vi "Queued State Machine.vi"() -> ()   [LabVIEW 2009]
doc: "Ce VI est un modèle de machine à états basée sur une file d'attente. Remplacez Processus 1 et Processus 2 par vos états. Pour ajouter d'autres processus, modifiez la constante énumération à définition de type. L'ordre de l'énumération doit correspondre à celui du cluster."
uses:
  Queued State Enum.ctl
panel:
  in  "Menu":T1
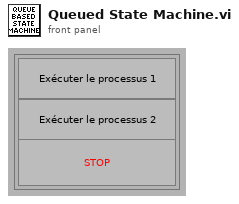
[diagram p1: front panel]
types:
  T1 = cluster{"Processus 1":bool, "Processus 2":bool, "stop":bool}
  T2 = typedef "Queued State Enum.ctl" = enum32{"Inactif", "Processus 1", "Processus 2", "Arrêt"}
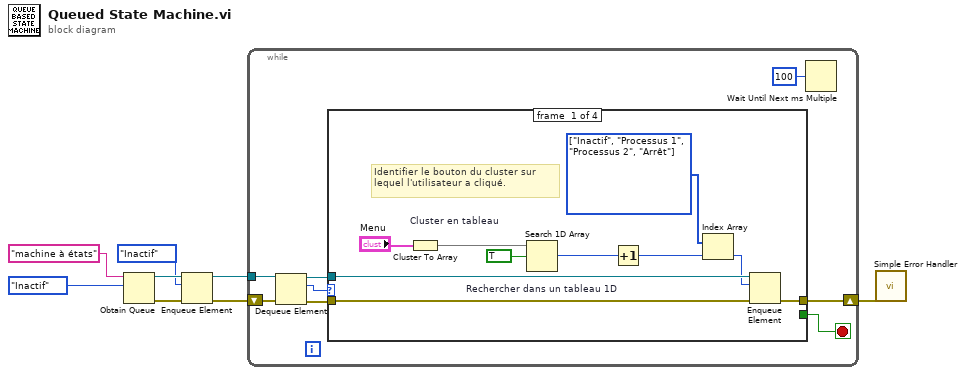
[diagram p0: block diagram]
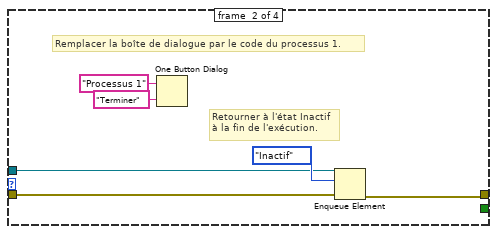
[diagram p2: hidden frame]
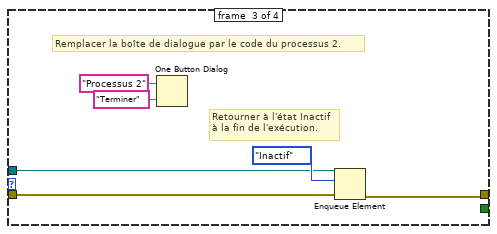
[diagram p3: hidden frame]
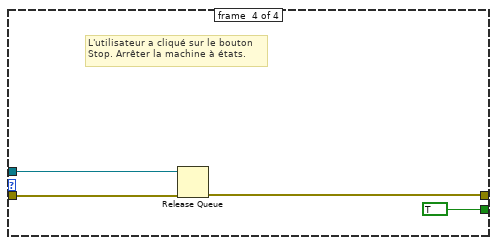
[diagram p4: hidden frame]
diagram:
  n1 = Obtain Queue ("Obtenir une file d'attente")(name (unnamed)="machine à états", element data type=Queued_State_Enum."Inactif" ("Enum")) -> (queue out=w6:refnum<queue>, error out=w7:errorcluster)  [unwired: 3 in, 1 out]
  n2 = Enqueue Element ("Ajouter un élément à la fin d'une file d'attente")(queue=w6, element=Queued_State_Enum."Inactif" ("Enum"), error in (no error)=w7) -> (queue out=w4:refnum<queue>, error out=w5:errorcluster)  [unwired: 2 out]
  n3 = while "Boucle While" {
    tunnel: w4 -> [w11]
    shift-right: [w14] -> w1
    shift-left: w5 -> [w13]
    stop <- w16 stop-if-true
    n4 = Dequeue Element ("Supprimer le premier élément d'une file d'attente")(queue=w11, error in (no error)=w13) -> (queue out=w10:refnum<queue>, element=w9:T2, error out=w12:errorcluster)  [unwired: 2 out]
    n5 = case "Structure Condition" shown="\"Inactif\", Par défaut" w9 {
      tunnel: [_ _ _ TRUE] -> w16
      tunnel: w12 -> [w22 w30 w36 w41]
      tunnel: w10 -> [w21 w27 w33 w40]
      tunnel: [w20 w29 w35 w39] -> w14
      frame #0 {
        w18 = T2[] [enum."Inactif", enum."Processus 1", enum."Processus 2", enum."Arrêt"] items=["Inactif", "Processus 1", "Processus 2", "Arrêt"]
        # "Identifier le bouton du cluster sur lequel l'utilisateur a cliqué."
        n6 = Cluster To Array "Cluster en tableau"(cluster="Menu") -> (array=w25:bool[])
        n7 = Search 1D Array "Rechercher dans un tableau 1D"(1D array=w25, element=TRUE) -> (index of element=w23:i32)  [unwired: 1 in]
        n8 = Increment(x=w23) -> (x+1=w19:i32)
        n9 = Index Array(array=w18, index=w19) -> (element=w17:T2)
        n10 = Enqueue Element(queue=w21, element=w17, error in (no error)=w22) -> (error out=w20:errorcluster)  [unwired: 3 out]
      }
      frame #1 {
        # "Retourner à l'état Inactif\nà la fin de l'exécution."
        # "Remplacer la boîte de dialogue par le code du processus 1."
        n11 = One Button Dialog(message="Processus 1", button name ("OK")="Terminer") -> ()  [unwired: 1 out]
        n12 = Enqueue Element(queue=w27, element=Queued_State_Enum."Inactif" ("Enum"), error in (no error)=w30) -> (error out=w29:errorcluster)  [unwired: 3 out]
      }
      frame #2 {
        # "Retourner à l'état Inactif\nà la fin de l'exécution."
        # "Remplacer la boîte de dialogue par le code du processus 2."
        n13 = One Button Dialog(message="Processus 2", button name ("OK")="Terminer") -> ()  [unwired: 1 out]
        n14 = Enqueue Element(queue=w33, element=Queued_State_Enum."Inactif" ("Enum"), error in (no error)=w36) -> (error out=w35:errorcluster)  [unwired: 3 out]
      }
      frame #3 {
        # "L'utilisateur a cliqué sur le bouton\nStop. Arrêter la machine à états."
        n15 = Release Queue(queue=w40, error in (no error)=w41) -> (error out=w39:errorcluster)  [unwired: 1 in, 2 out]
      }
    }
    n16 = Wait Until Next ms Multiple ("Attendre un multiple de ms")(millisecond multiple=u32 100) -> ()  [unwired: 1 out]
  }
  n17 = call <vilib>:"Simple Error Handler.vi"("error in (no error)"=w1) -> ()  [unwired: 1 in, 8 out]
